vi "Set board image.vi"(8 "error in (no error)":errorcluster, 10 "board image":T1, 11 "Assembly Line Input in":refnum<class "Assembly Line Input.lvclass">) -> (0 "error out":errorcluster, 3 "Assembly Line Input out":refnum<class "Assembly Line Input.lvclass">)   [LabVIEW 2018, in "Assembly Line Input.lvclass"]
uses:
  Assembly Line Input.lvclass
  Common/Board Image.ctl
  Assembly Line Input.lvclass/Assembly Line Input.ctl
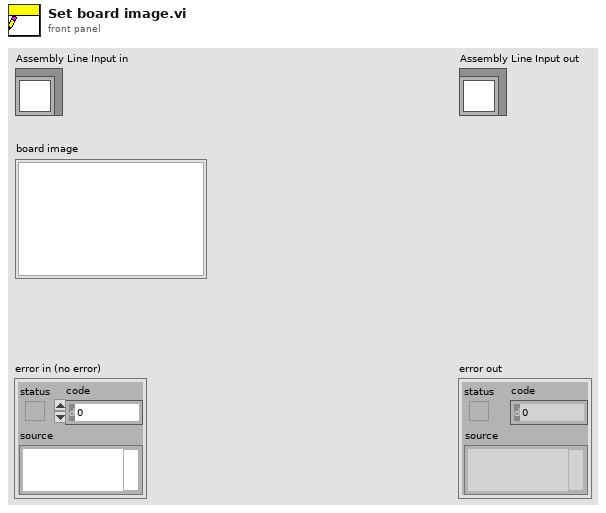
[diagram p1: front panel]
types:
  T1 = typedef "Board Image.ctl" = picture
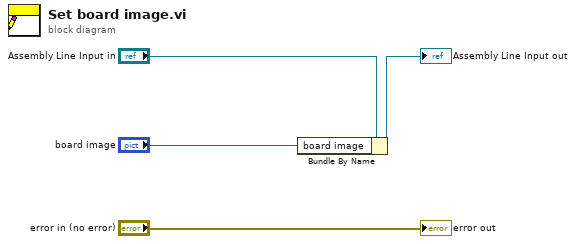
[diagram p0: block diagram]
diagram:
  n1 = Bundle By Name(cluster="Assembly Line Input in", "board image"="board image") -> (→"Assembly Line Input out":refnum<class "Assembly Line Input.lvclass">)
  "error out" <- "error in (no error)"
